vi "Trigger--Const.vi"() -> (3 "Trigger Command":string)   [LabVIEW 2017, in "Communications Library.lvlib"]
uses:
  Communications Library.lvlib
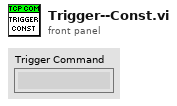
[diagram p1: front panel]
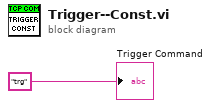
[diagram p0: block diagram]
diagram:
  "Trigger Command" <- "trg" ("data in")
